vi "PointInTri.vi"(9 "v":dbl[](array[numeric]), 10 "u":dbl[](array[numeric]), 11 "w":dbl[](array[numeric])) -> (3 "PointInTri":bool)   [LabVIEW 2014]
uses:
  <vilib>/Analysis/baseanly.llb/Real Dot Product.vi
  <vilib>/Analysis/NI_AALBase.lvlib
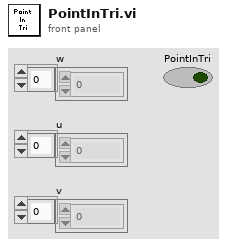
[diagram p1: front panel]
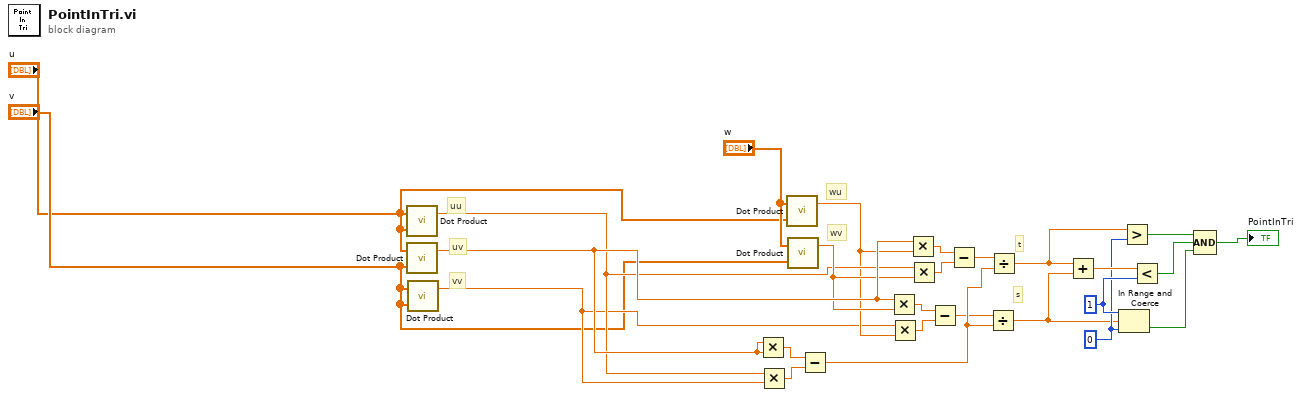
[diagram p0: block diagram]
diagram:
  w21 = 1
  w19 = 0
  # "t"
  # "s"
  # "wv"
  # "wu"
  # "vv"
  # "uv"
  # "uu"
  n1 = call-poly <vilib>:"Dot Product.vi"("Y Vector"="u", "X Vector"="u") -> ("X * Y"=w13:dbl)  [unwired: 1 out]
  n2 = call-poly <vilib>:"Dot Product.vi"("Y Vector"="v", "X Vector"="u") -> ("X * Y"=w26:dbl)  [unwired: 1 out]
  n3 = call-poly <vilib>:"Dot Product.vi"("Y Vector"="v", "X Vector"="v") -> ("X * Y"=w6:dbl)  [unwired: 1 out]
  n4 = Multiply(x=w26, y=w26) -> (x*y=w4:dbl)
  n5 = Multiply(x=w13, y=w6) -> (x*y=w5:dbl)
  n6 = call-poly <vilib>:"Dot Product.vi"("Y Vector"="u", "X Vector"="w") -> ("X * Y"=w12:dbl)  [unwired: 1 out]
  n7 = call-poly <vilib>:"Dot Product.vi"("Y Vector"="v", "X Vector"="w") -> ("X * Y"=w14:dbl)  [unwired: 1 out]
  n8 = Subtract(x=w4, y=w5) -> (x-y=w16:dbl)
  n9 = Multiply(x=w26, y=w14) -> (x*y=w7:dbl)
  n10 = Multiply(x=w6, y=w12) -> (x*y=w8:dbl)
  n11 = Multiply(x=w26, y=w12) -> (x*y=w11:dbl)
  n12 = Multiply(x=w13, y=w14) -> (x*y=w10:dbl)
  n13 = Subtract(x=w7, y=w8) -> (x-y=w9:dbl)
  n14 = Subtract(x=w11, y=w10) -> (x-y=w15:dbl)
  n15 = Divide(x=w9, y=w16) -> (x/y=w17:dbl)
  n16 = Divide(x=w15, y=w16) -> (x/y=w18:dbl)
  n17 = Add(x=w18, y=w17) -> (x+y=w20:dbl)
  n18 = In Range and Coerce(upper limit=w21, x=w17, lower limit=w19) -> (In Range?=w24:bool)  [unwired: 1 out]
  n19 = Greater?(x=w18, y=w19) -> (0:w22:bool)
  n20 = Less?(x=w20, y=w21) -> (x < y?=w23:bool)
  n21 = Compound Arithmetic op=AND(w22, w23, w24) -> (→"PointInTri":bool)
